vi "Generate Bounds Coordinates.vi"(1 "Height":u32, 2 "Width":u32) -> (0 "bounds":T1)   [LabVIEW 2019, in "gRPC Template Creation Utility.lvlib"]
uses:
  gRPC Template Creation Utility.lvlib
  <vilib>/Utility/miscctls.llb/LVBoundsTypeDef.ctl
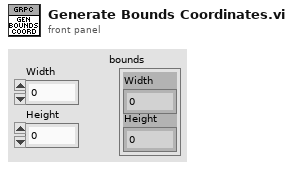
[diagram p1: front panel]
types:
  T1 = typedef "LVBoundsTypeDef.ctl" = cluster{"Width":u32, "Height":u32}
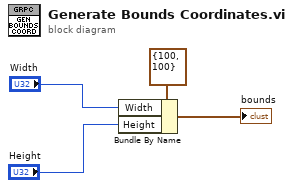
[diagram p0: block diagram]
diagram:
  n1 = Bundle By Name(cluster=T1 {"Width"=100, "Height"=100} ("bounds"), "Width"="Width", "Height"="Height") -> (→"bounds":T1)
